vi "Main v0.86.vi"() -> ()   [LabVIEW 2017]
doc: "v0.85:\n- Counts for rejects and total\n\nv0.5:\n\n- Added Reject to Manual Mode\n- Send reject pallet cluster during manual mode\n- Run continuous manual happens only when no error has occured"
uses:
  Controls/Main Tabs.ctl
  Controls/Auto.ctl
  RT/Controls/Auto Delays.ctl
  RT/Controls/Auto Times.ctl
  Controls/UI Data.ctl
  support/Message Queue/Enqueue Message (Single).vi
  <vilib>/Utility/error.llb/Error Cluster From Error Code.vi
  <vilib>/ErrorRing/Error Ring.xnode
  support/Message Queue/Message Queue.lvlib
  support/User Event - Stop/User Event - Stop.lvlib
panel:
  in  "Reject Pallets":T1
  out "Date-Time":string caption="Dip-Tube Assembly Automation (HMI) v0.85"
  out "Main Tab":T2
  in  "Autocycle":T3
  in  "Manual":bool
  in  "Parameters":bool
  in  "Maintenance":bool
  in  "Save Para":bool
  in  "Home Para":bool
  in  "ParaTab":T4(tab)
  in  "StopperRearDelay":dbl format="%#.2f"
  in  "StopperFrontDelay":dbl format="%#.2f"
  in  "MaxAlarms":dbl caption="Max Alarms in 1 Minute" format="%#.2f"
  in  "MaxConsecutive":dbl caption="Max Consecutive Alarms" format="%#.2f"
  in  "Gate Close Delay":dbl format="%#.2f"
  in  "Gate Open Delay":dbl format="%#.2f"
  in  "BF Off Delay":dbl format="%#.2f"
  in  "BF On Delay":dbl format="%#.2f"
  in  "DelayAfterReject":dbl format="%#.2f"
  in  "MeasurementTime":dbl format="%#.2f"
  in  "DelayAfterMesFront":dbl format="%#.2f"
  in  "DelayAfterCut":dbl format="%#.2f"
  in  "DelayAfterCutClamp":dbl format="%#.2f"
  in  "DelayAfterInsClamp":dbl format="%#.2f"
  in  "DelayToClose":dbl format="%#.2f"
  in  "DelayToOpen":dbl format="%#.2f"
  in  "DelayAfterInsertion":dbl format="%#.2f"
  in  "DelayBeforeInsertion":dbl format="%#.2f"
  in  "AgitatorUpTime":dbl format="%#.2f"
  in  "AgitatorDownTime":dbl format="%#.2f"
  out "OEE":dbl format="%#.1f"
  out "QUA":dbl=100.0 min=0.0 max=100.0 step=0.1
  in  "Ideal Time":dbl=2.0 min=0.0 max=100.0 step=0.1
  in  "AVL":dbl=100.0 min=0.0 max=100.0 step=0.1
  out "Rejects":u32
  in  "Reset MCount":bool
  in  "Enable BF?":bool
  in  "Enable Agitate?":bool
  in  "Enable Reject?":bool
  in  "Toggle Motor":bool
  in  "Continuous?":bool
  in  "Enable Measure?":bool
  in  "Enable Index?":bool
  in  "Enable PF?":bool
  in  "Auto Delays":T5={"Agitator Delays"=[400, 250], "TF Delays"=[700, 800, 2], "Insertion Delays"=[100, 500], "Cutting Delays"=[300, 300, 100], "PF Delays"=[250, 30000], "Measur. Delays"=[500.0, 188.9, 1.0], "Reject Delays"=[500], "BF Delays"=[1000, 1000]}
  in  "Enable Cutting?":bool
  in  "Enable Insertion?":bool
  in  "Run Manual":bool
  in  "Enable TF?":bool
  in  "Home Manual":bool
  out "Status":T7
  out "Measurements":T8 {"Height 1" format="%#.2f"; "Height 2" format="%#.2f"; "Height 3" format="%#.2f"; "Height 4" format="%#.2f"}
  out "Output Count":u32 caption="Output\nCount"
  out "PRF":dbl=100.0 min=0.0 max=100.0 step=0.1
  in  "All IO":bool
  in  "Stats":bool
  in  "Home AC":bool
  out "Status":string
  out "Count":dbl format="%06.0f"
  out "Count 3":dbl caption="Cycle Time" format="%0.2f"
  out "Count 2":dbl caption="Rejects" format="%06.0f"
  in  "Statuses":string[][](table)
  in  "Exit":bool
  # "Vision Harmony Dip-Tube Assembly Automation"
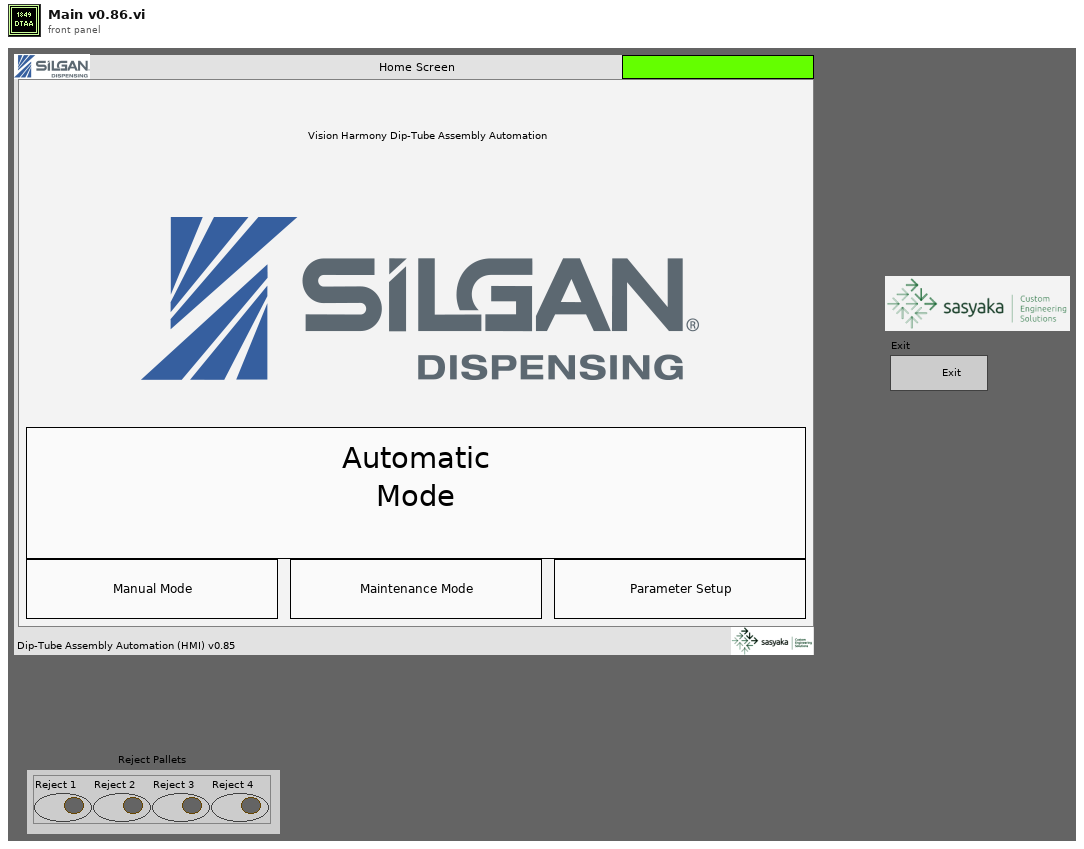
[diagram p1: front panel]
types:
  T1 = cluster{"Reject 1":bool, "Reject 2":bool, "Reject 3":bool, "Reject 4":bool}
  T2 = typedef "Main Tabs.ctl" = enum32{"Home Screen", "Parameter Setup", "Manual Mode", "Autocycle"}
  T3 = typedef "Auto.ctl" = bool
  T4 = enum32{"General & Indexing", "Bowl Feeder & Pump Conveyor", "Cutting, Measurement & Rejection", "Tube Feeder & Insertion"}
  T5 = typedef "Auto Delays.ctl" = cluster{"Agitator Delays":u32[], "TF Delays":u32[], "Insertion Delays":u32[], "Cutting Delays":u32[], "PF Delays":u32[], "Measur. Delays":dbl[], "Reject Delays":u32[], "BF Delays":u32[]}
  T6 = typedef "Auto Times.ctl" = cluster{"Index Time":u32, "TF Time":u32, "Insertion Time":u32, "Cutting Time":u32, "PF Time":u32, "Meas. Time":u32, "Reject Time":u32}
  T7 = cluster{"Auto Times":T6, "error out":errorcluster}
  T8 = cluster{"Height 1":dbl, "Height 2":dbl, "Height 3":dbl, "Height 4":dbl}
  T9 = typedef "UI Data.ctl" = cluster{"Main Tab":refnum<vi>}
  T10 = typedef "Message Queue.lvlib/All Message Queues.ctl" = cluster{"UI":refnum<queue>}
  T11 = enum8{"Enabled", "Disabled", "Disabled and Grayed Out"}
  T12 = cluster{"Auto Times":T6, "Results":cluster{"Measurements":cluster{"1":dbl, "2":dbl, "3":dbl, "4":dbl}, "Reject Pallets":cluster{"Reject 1":bool, "Reject 2":bool, "Reject 3":bool, "Reject 4":bool}}, "OutputCount":u32, "error out":errorcluster}
  T13 = cluster{"Auto Delays":T5, "Reject Pallets":cluster{"Reject 1":bool, "Reject 2":bool, "Reject 3":bool, "Reject 4":bool}}
  T14 = cluster{"Measurements":cluster{"1":dbl, "2":dbl, "3":dbl, "4":dbl}, "Reject Pallets":cluster{"Reject 1":bool, "Reject 2":bool, "Reject 3":bool, "Reject 4":bool}}
  T15 = cluster{"AVL":dbl, "PRF":dbl, "QUA":dbl, "OEE":dbl}
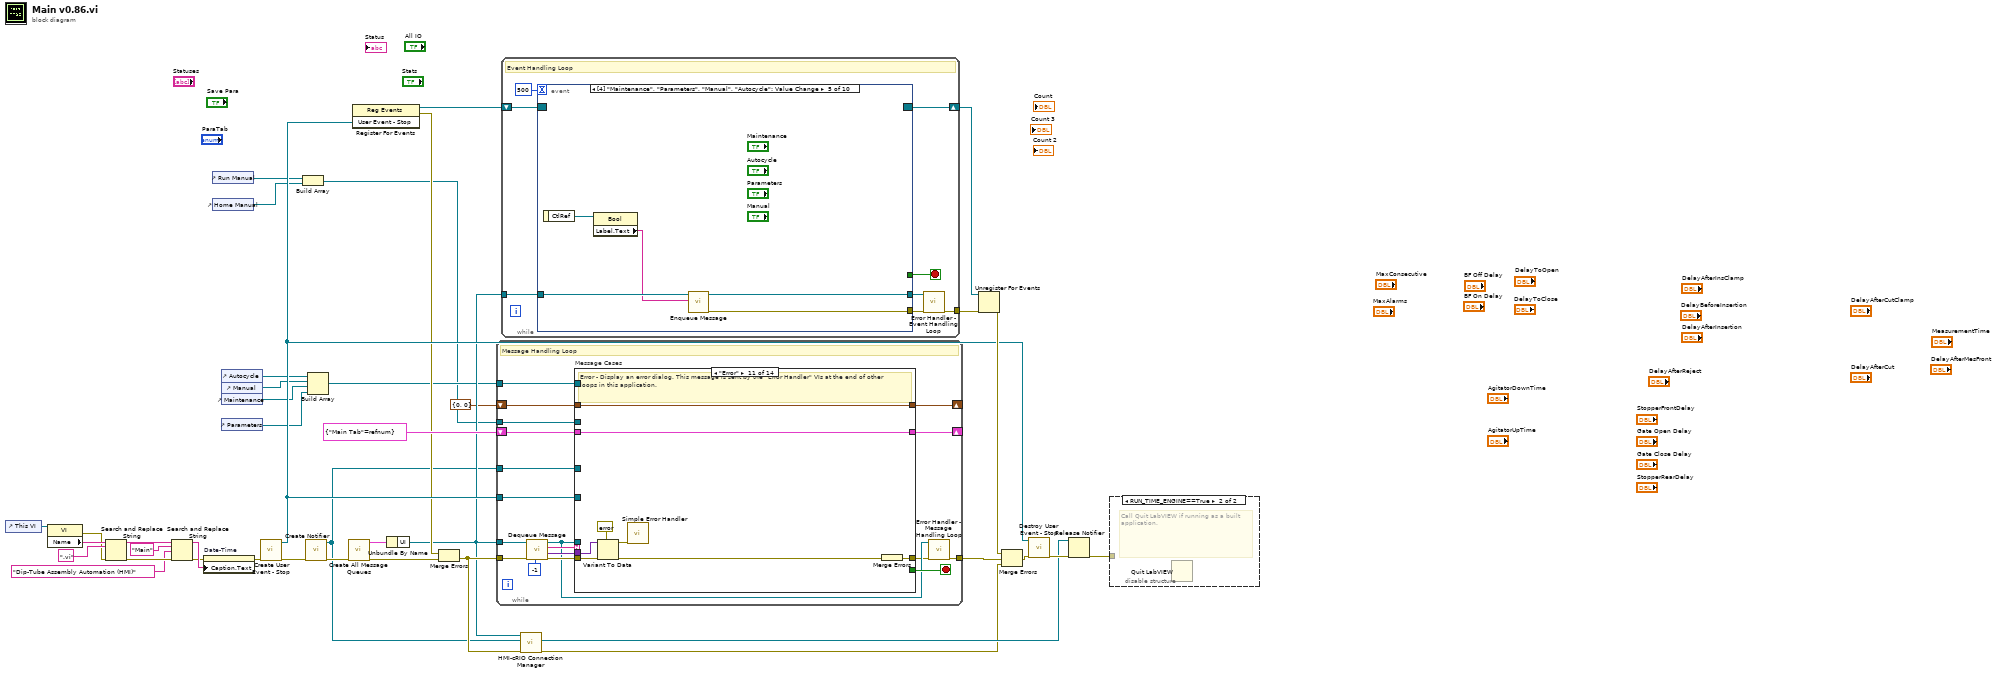
[diagram p0: block diagram]
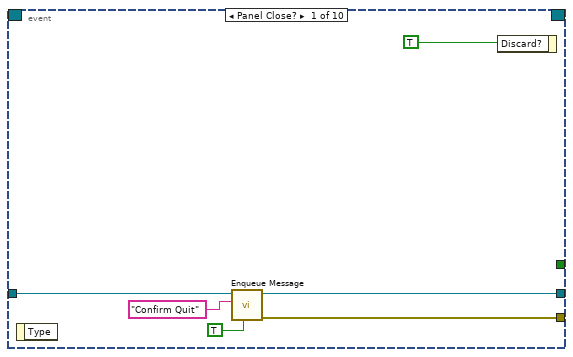
[diagram p2: hidden frame]
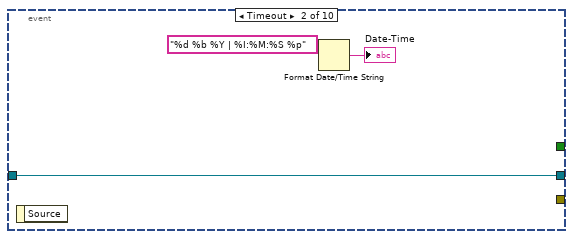
[diagram p3: hidden frame]
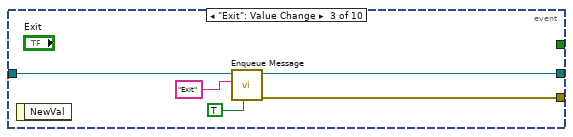
[diagram p4: hidden frame]
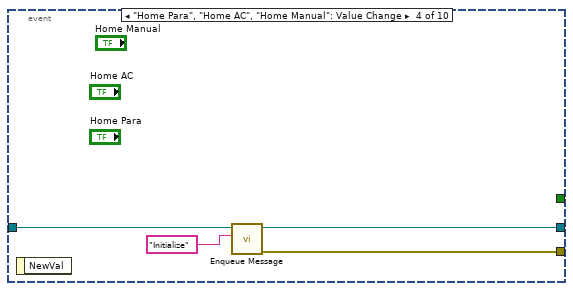
[diagram p5: hidden frame]
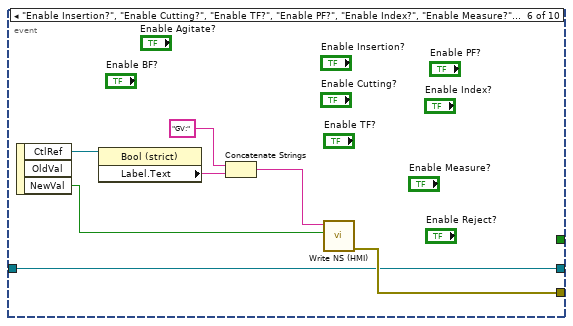
[diagram p6: hidden frame]
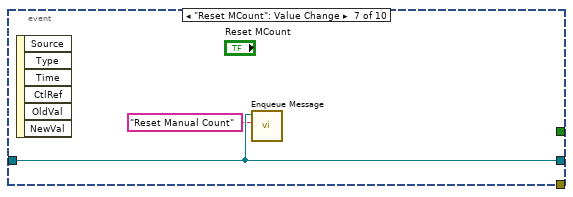
[diagram p7: hidden frame]
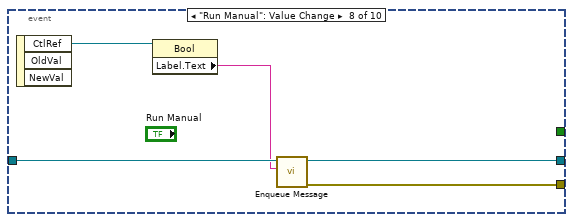
[diagram p8: hidden frame]
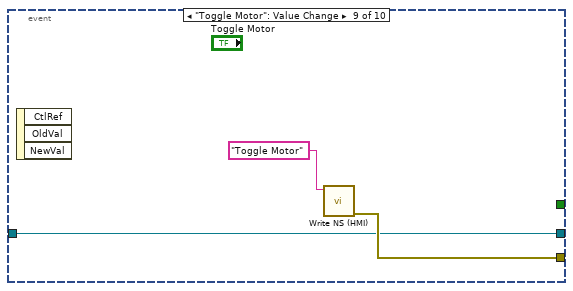
[diagram p9: hidden frame]
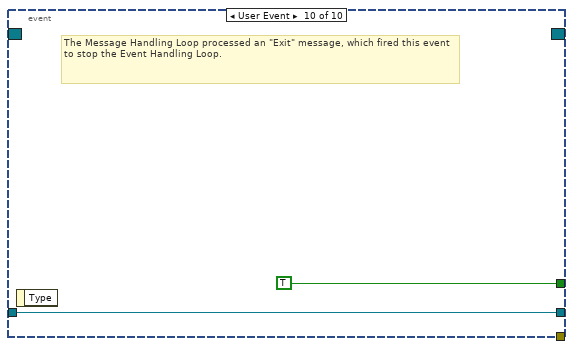
[diagram p10: hidden frame]
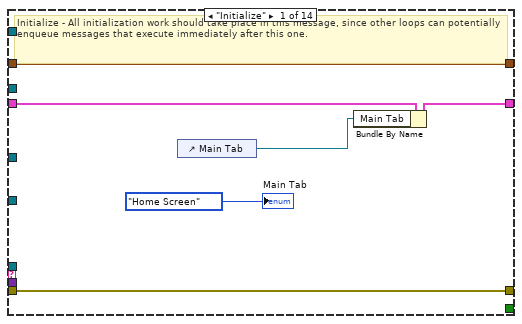
[diagram p11: hidden frame]
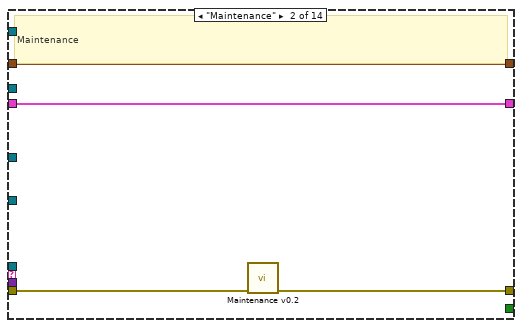
[diagram p12: hidden frame]
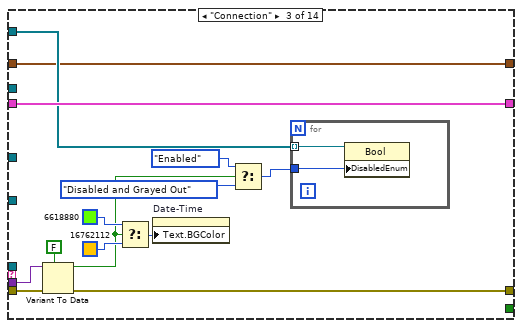
[diagram p13: hidden frame]
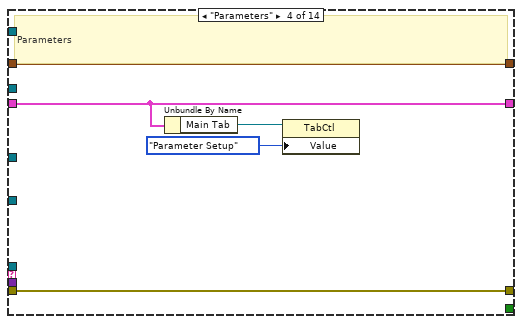
[diagram p14: hidden frame]
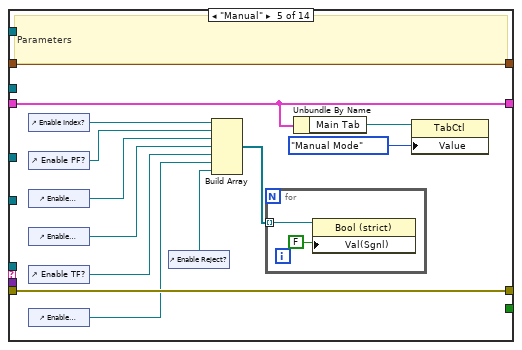
[diagram p15: hidden frame]
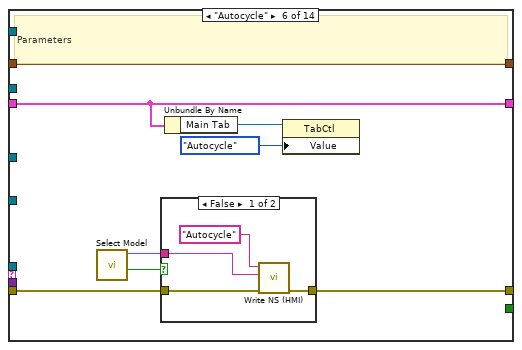
[diagram p16: hidden frame]
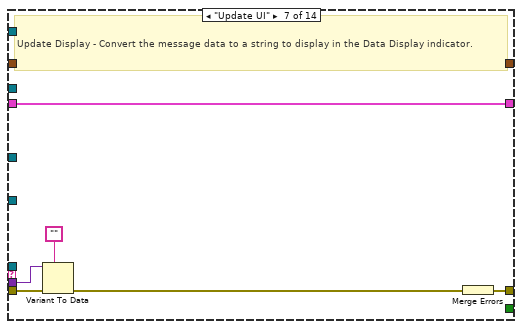
[diagram p18: hidden frame]
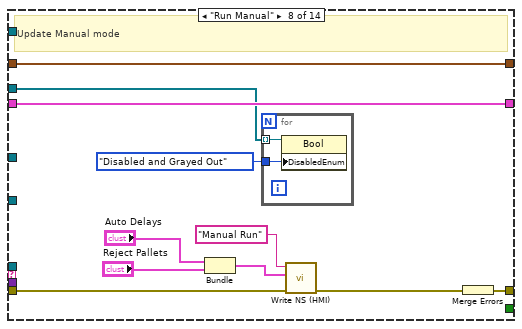
[diagram p19: hidden frame]
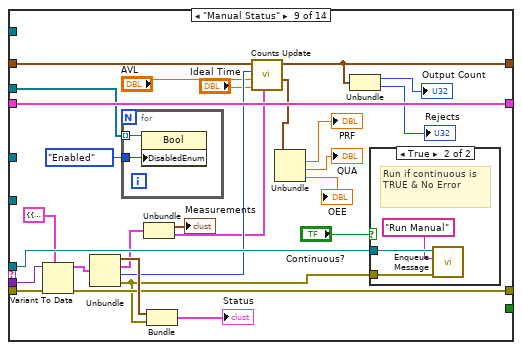
[diagram p20: hidden frame]
diagram:
  n1 = control-ref of="This VI"() -> (w9:refnum<vi>)
  n2 = property class="VI"(reference=w9) -> (error out=w8:errorcluster, "Name"=w15:string)  [unwired: 1 in, 1 out]
  n3 = Search and Replace String(input string=w15, search string=".vi", error in=w8) -> (result string=w13:string, error out=w12:errorcluster)  [unwired: 5 in, 2 out]
  n4 = Search and Replace String(input string=w13, search string="Main", replace string="Dip-Tube Assembly Automation (HMI)" ("replace string (\"\")"), error in=w12) -> (result string=w7:string, error out=w6:errorcluster)  [unwired: 4 in, 2 out]
  n5 = property on="Date-Time" class="Str"(error in=w6, "Caption.Text"=w7) -> (error out=w5:errorcluster)  [unwired: 1 in, 1 out]
  n6 = control-ref of="Run Manual"() -> (w4:refnum<vi>)
  n7 = control-ref of="Home Manual"() -> (w3:refnum<vi>)
  n8 = control-ref of="Autocycle"() -> (w20:refnum<vi>)
  n9 = control-ref of="Manual"() -> (w19:refnum<vi>)
  n10 = control-ref of="Maintenance"() -> (w18:refnum<vi>)
  n11 = control-ref of="Parameters"() -> (w17:refnum<vi>)
  n12 = call "Create User Event - Stop.vi"("error in (no error)"=w5) -> ("error out"=w27:errorcluster, "User Event - Stop"=w31:refnum<user-event>)  [unwired: 9 in]
  n13 = Build Array(w4, w3) -> (w2:refnum<vi>[])
  n14 = call "Create Notifier.vi"("error in (no error)"=w27) -> ("error out"=w26:errorcluster, "notifier out"=w21:refnum<notifier>)  [unwired: 9 in]
  n15 = Build Array(w20, w19, w18, w17) -> (w16:refnum<vi>[])
  n16 = call "Create All Message Queues.vi"("error in (no error)"=w26) -> ("error out"=w40:errorcluster, "Message Queues out"=w39:T10)  [unwired: 9 in]
  n17 = register-events(w31) -> (reference out=w32:refnum<event-registration>, error out=w30:errorcluster)  [unwired: 2 in]
  n18 = Unbundle By Name(w39) -> ("UI"=w28:refnum<queue>)
  n19 = Merge Errors(w30, w40) -> (w29:errorcluster)
  n20 = while {
    tunnel: w28 -> [w50]
    shift-right: [w57] -> _
    shift-left: T9 {"Main Tab"=refnum} ("Data Cluster") -> [w58]
    tunnel: w31 -> [w55]
    tunnel: w29 -> [w54]
    tunnel: [w48] -> w38
    tunnel: w21 -> [w45]
    tunnel: w16 -> [w44]
    tunnel: w2 -> [w43]
    shift-right: [w41] -> _
    shift-left: cluster{"OutputCount":u32, "RejectCount":u32} {"OutputCount"=0, "RejectCount"=0} -> [w42]
    stop <- w56 stop-if-true
    # "Message Handling Loop"
    n21 = call "Dequeue Message.vi"("timeout"=-1, "error in (no error)"=w54, "Message Queue"=w50) -> ("error out"=w53:errorcluster, "Message Data"=w51:variant, "Message"=w52:string, "dup Message Queue"=w49:refnum<queue>)  [unwired: 5 in]
    n22 = case "Message Cases" shown="\"Error\"" w52 {
      selector: w52 -> [_ _ _ _ _ _ _ _ _ _ _ _ _ w206]
      tunnel: w49 -> [_ _ _ _ _ _ _ _ w155 _ _ w185 w204 _]
      tunnel: w53 -> [w64 w67 w80 w89 w102 w108 w122 w132 w163 w173 w181 w189 w197 _]
      tunnel: [w64 w66 w79 w89 w102 w107 w123 w134 w154 w173 w175 w187 w200 w207] -> w47
      tunnel: w58 -> [w63 w68 w82 w88 w101 w112 w124 w135 w164 w172 w180 w188 w203 w208]
      tunnel: [w62 w68 w82 w88 w101 w112 w124 w135 w164 w172 w180 w188 w203 w208] -> w57
      tunnel: [_ _ _ _ _ _ _ _ _ _ _ _ TRUE _] -> w56
      tunnel: w51 -> [_ _ w78 _ _ _ w121 _ w162 _ w179 _ w194 _]
      tunnel: w55 -> [_ _ _ _ _ _ _ _ _ _ _ _ w199 _]
      tunnel: w45 -> [_ _ _ _ _ _ _ _ _ _ _ _ w193 _]
      tunnel: w44 -> [_ _ w74 _ _ _ _ _ _ _ _ _ _ _]
      tunnel: w43 -> [_ _ _ _ _ _ _ w129 w160 _ _ _ _ _]
      tunnel: w42 -> [w59 w65 w69 w85 w90 w109 w118 w125 w153 _ w174 w182 w190 w205]
      tunnel: [w59 w65 w69 w85 w90 w109 w118 w125 w146 cluster{"OutputCount":u32, "RejectCount":u32} {"OutputCount"=0, "RejectCount"=0} w174 w182 w190 w205] -> w41
      frame "Initialize" {
        # "Initialize - All initialization work should take place in this message, since other loops can potentially enqueue messages that execute immediately after this one."
        n23 = control-ref of="Main Tab"() -> (w61:refnum<vi>)
        n24 = Bundle By Name(cluster=w63, "Main Tab"=w61) -> (w62:T9)
        "Main Tab" <- Main_Tabs."Home Screen" ("Main Tab")
      }
      frame "Maintenance" {
        # "Maintenance"
        n25 = call "Maintenance v0.2.vi"("Error In"=w67) -> ("Error out"=w66:errorcluster)  [unwired: 10 in]
      }
      frame "Connection" {
        n26 = Variant To Data(error in=w80, type=FALSE, Variant=w78) -> (data=w73:bool, error out=w79:errorcluster)
        n27 = Select(t=u32 6618880 ("Text.Text Colors:BG Color"), s=w73, f=u32 16762112 ("Text.Text Colors:BG Color")) -> (s? t:f=w75:u32)
        n28 = property on="Date-Time" class="Str"("Text.BGColor"=w75) -> ()  [unwired: 2 in, 2 out]
        n29 = Select(t=T11."Enabled" ("Disabled"), s=w73, f=T11."Disabled and Grayed Out") -> (s? t:f=w71:T11)
        n30 = for {
          tunnel: w74 -> [w84] mode=indexing
          tunnel: w71 -> [w83]
          n31 = property class="Bool"(reference=w84, "DisabledEnum"=w83) -> ()  [unwired: 1 in, 2 out]
        }
      }
      frame "Parameters" {
        # "Parameters"
        n32 = Unbundle By Name(w88) -> ("Main Tab"=w87:refnum<vi>)
        n33 = property class="TabCtl"(reference=w87, "Value"=Main_Tabs."Parameter Setup" ("Main Tab")) -> ()  [unwired: 1 in, 2 out]
      }
      frame "Manual" {
        # "Parameters"
        n34 = control-ref of="Enable Index?"() -> (w98:refnum<vi>)
        n35 = control-ref of="Enable PF?"() -> (w97:refnum<vi>)
        n36 = control-ref of="Enable Cutting?"() -> (w96:refnum<vi>)
        n37 = control-ref of="Enable Insertion?"() -> (w95:refnum<vi>)
        n38 = control-ref of="Enable TF?"() -> (w94:refnum<vi>)
        n39 = control-ref of="Enable Measure?"() -> (w92:refnum<vi>)
        n40 = control-ref of="Enable Reject?"() -> (w91:refnum<vi>)
        n41 = Build Array(w98, w97, w96, w95, w94, w92, w91) -> (w93:refnum<vi>[])
        n42 = for {
          tunnel: w93 -> [w104] mode=indexing
          n43 = property class="Bool (strict)"(reference=w104, "Val(Sgnl)"=FALSE ("Value (Signaling)")) -> ()  [unwired: 1 in, 2 out]
        }
        n44 = Unbundle By Name(w101) -> ("Main Tab"=w100:refnum<vi>)
        n45 = property class="TabCtl"(reference=w100, "Value"=Main_Tabs."Manual Mode" ("Main Tab")) -> ()  [unwired: 1 in, 2 out]
      }
      frame "Autocycle" {
        # "Parameters"
        n46 = call "Select Model.vi"() -> ("Cancel out"=w105:bool, "Model out"=w106:string)  [unwired: 10 in]
        n47 = case shown="False" w105 {
          tunnel: w108 -> [w115 w117]
          tunnel: [w114 w117] -> w107
          tunnel: w106 -> [w113 _]
          frame False {
            n48 = call "Write NS (HMI).vi"("error in (no error)"=w115, "Message Data"=w113, "Message"="Autocycle") -> ("error out"=w114:errorcluster)  [unwired: 8 in]
          }
          frame True {
          }
        }
        n49 = Unbundle By Name(w112) -> ("Main Tab"=w111:refnum<vi>)
        n50 = property class="TabCtl"(reference=w111, "Value"=Main_Tabs."Autocycle" ("Main Tab")) -> ()  [unwired: 1 in, 2 out]
      }
      frame "Update UI" {
        # "Update Display - Convert the message data to a string to display in the Data Display indicator."
        n51 = Variant To Data(error in=w122, type="", Variant=w121) -> (error out=w119:errorcluster)  [unwired: 1 out]
        n52 = Merge Errors(w119) -> (w123:errorcluster)
      }
      frame "Run Manual" {
        # "Update Manual mode"
        n53 = Bundle("Auto Delays"="Auto Delays", "Reject Pallets"="Reject Pallets") -> (w126:T13)  [unwired: 1 in]
        n54 = for {
          tunnel: w129 -> [w137] mode=indexing
          tunnel: T11."Disabled and Grayed Out" ("Disabled") -> [w136]
          n55 = property class="Bool"(reference=w137, "DisabledEnum"=w136) -> ()  [unwired: 1 in, 2 out]
        }
        n56 = call "Write NS (HMI).vi"("error in (no error)"=w132, "Message Data"=w126, "Message"="Manual Run") -> ("error out"=w131:errorcluster)  [unwired: 8 in]
        n57 = Merge Errors(w131) -> (w134:errorcluster)
      }
      frame "Manual Status" {
        n58 = Variant To Data(error in=w163, type=T12 {"Auto Times"={"Index Time"=0, "TF Time"=0, "Insertion Time"=0, "Cutting Time"=0, "PF Time"=0, "Meas. Time"=0, "Reject Time"=0}, "Results"={"Measurements"={"1"=0.0, "2"=0.0, "3"=0.0, "4"=0.0}, "Reject Pallets"={"Reject 1"=FALSE, "Reject 2"=FALSE, "Reject 3"=FALSE, "Reject 4"=FALSE}}, "OutputCount"=0, "error out"={"status"=FALSE, "code"=0, "source"=""}} ("cluster"), Variant=w162) -> (data=w159:T12, error out=w154:errorcluster)
        n59 = Unbundle(w159) -> ("Auto Times"=w158:T6, "Results"=w150:T14, "OutputCount"=w148:u32, "error out"=w152:errorcluster)
        n60 = for {
          tunnel: w160 -> [w169] mode=indexing
          tunnel: T11."Enabled" ("Disabled") -> [w168]
          n61 = property class="Bool"(reference=w169, "DisabledEnum"=w168) -> ()  [unwired: 1 in, 2 out]
        }
        n62 = Unbundle(w150) -> ("Measurements"=→"Measurements":cluster{"1":dbl, "2":dbl, "3":dbl, "4":dbl}, "Reject Pallets"=w147:T1)
        n63 = Bundle("Auto Times"=w158, "error out"=w152) -> (→"Status":T7)  [unwired: 1 in]
        n64 = call "Counts Update.vi"("Reject Pallets"=w147, "Desired Cycle Time"="Ideal Time", "AVL"="AVL", "OutputCount"=w148, "Counts in"=w153) -> ("OEE"=w141:T15, "Counts out"=w146:cluster{"OutputCount":u32, "RejectCount":u32})  [unwired: 5 in]
        n65 = Unbundle(w141) -> ("PRF"=→"PRF":dbl, "QUA"=→"QUA":dbl, "OEE"=→"OEE":dbl)  [unwired: 1 out]
        n66 = Unbundle(w146) -> ("OutputCount"=→"Output Count":u32, "RejectCount"=→"Rejects":u32)
        n67 = case shown="True" "Continuous?" {
          tunnel: w155 -> [_ w167]
          tunnel: w152 -> [_ w166]
          frame False {
          }
          frame True {
            # "Run if continuous is TRUE & No Error"
            n68 = call-poly "Enqueue Message.vi"("error in (no error)"=w166, "Message"="Run Manual", "Message Queue"=w167) -> ()  [unwired: 7 in, 2 out]
          }
        }
      }
      frame "Reset Manual Count" {
        w170 = u32 0 ("Rejects")
        n69 = local write "Output Count"(w170) -> ()
        n70 = local write "Rejects"(w170) -> ()
      }
      frame "Error" {
        # "Error - Display an error dialog. This message is sent by the \"Error Handler\" VIs at the end of other loops in this application."
        n71 = Variant To Data(error in=w181, type=errorcluster {"status"=FALSE, "code"=0, "source"=""} ("error constant"), Variant=w179) -> (data=w177:errorcluster, error out=w176:errorcluster)
        n72 = call <vilib>:"Simple Error Handler.vi"("error in (no error)"=w177) -> ()  [unwired: 4 in, 5 out]
        n73 = Merge Errors(w176) -> (w175:errorcluster)
      }
      frame "Confirm Quit" {
        # "Confirm Quit - Message that can confirm whether or not the user wants to exit the application."
        n74 = call-poly "Enqueue Message.vi"("Priority Message? (F)"=TRUE, "error in (no error)"=w189, "Message"="Exit", "Message Queue"=w185) -> ("error out"=w186:errorcluster)  [unwired: 6 in, 1 out]
        n75 = Merge Errors(w186) -> (w187:errorcluster)
      }
      frame "Exit" {
        # "Stop the VI"
        # "Release the message queue reference"
        # "Exit - Exit the application."
        n76 = Variant To Data(type=errorcluster {"status"=FALSE, "code"=0, "source"=""} ("error constant"), Variant=w194) -> (data=w195:errorcluster)  [unwired: 1 in, 1 out]
        n77 = call <vilib>:"Simple Error Handler.vi"("error in (no error)"=w195) -> ()  [unwired: 4 in, 5 out]
        n78 = Send Notification(notification=TRUE, notifier=w193) -> (error out=w191:errorcluster)  [unwired: 1 in, 1 out]
        n79 = call "Fire User Event - Stop.vi"("User Event - Stop"=w199) -> ("error out"=w198:errorcluster)  [unwired: 10 in]
        n80 = Release Queue(queue=w204, error in (no error)=w197) -> (error out=w201:errorcluster)  [unwired: 1 in, 2 out]
        n81 = Merge Errors(w191, w198, w201) -> (w200:errorcluster)
      }
      frame Default {
        # "'Default' case only runs if there is a message that isn't defined in any of the other cases.  Output a programming error."
        n82 = xnode "Error Ring"("parameter 0"=w206) -> ("error out"=w207:errorcluster)
      }
    }
    n83 = call "Error Handler - Message Handling Loop.vi"("error in (no error)"=w47, "Message Queue"=w49) -> ("dup error in"=w48:errorcluster)  [unwired: 8 in, 1 out]
  }
  n84 = while {
    tunnel: w28 -> [w223]
    shift-right: [w221] -> w35
    shift-left: w32 -> [w222]
    tunnel: [w217] -> w33
    stop <- w219 stop-if-true
    # "Event Handling Loop"
    n85 = event shown="[4] \"Maintenance\", \"Parameters\", \"Manual\", \"Autocycle\": Value Change" {
      selector: w222 -> [_ _ _ _ _ _ _ _ _ _]
      dyn-events: [_ _ _ _ _ _ _ _ _ _] -> w221
      timeout: 500 -> [_ _ _ _ _ _ _ _ _ _]
      tunnel: [_ _ _ _ _ _ _ _ _ TRUE ("Discard?")] -> w219
      tunnel: w223 -> [w228 w232 w237 w241 w246 w251 w255 w260 w262 w265]
      tunnel: [w227 _ w236 w240 w245 w252 _ w258 w263 _] -> w220
      tunnel: [w226 w232 w235 w239 w244 w251 w255 w259 w262 w265] -> w218
      event Panel Close? {
        n86 = event-data() -> ()  [unwired: 1 in, 1 out]
        n87 = call-poly "Enqueue Message.vi"("Priority Message? (F)"=TRUE, "Message"="Confirm Quit", "Message Queue"=w228) -> ("error out"=w227:errorcluster, "dup Message Queue"=w226:refnum<queue>)  [unwired: 7 in]
        n88 = event-data("Discard?"=TRUE) -> ()  [unwired: 1 in, 1 out]
      }
      event Timeout {
        n89 = event-data() -> ()  [unwired: 1 in, 1 out]
        n90 = Format Date/Time String(time format string (%c)="%d %b %Y | %I:%M:%S %p") -> (date/time string=→"Date-Time":string)  [unwired: 2 in]
      }
      event "Exit": Value Change {
        n91 = event-data() -> ()  [unwired: 1 in, 1 out]
        n92 = call-poly "Enqueue Message.vi"("Priority Message? (F)"=TRUE, "Message"="Exit", "Message Queue"=w237) -> ("error out"=w236:errorcluster, "dup Message Queue"=w235:refnum<queue>)  [unwired: 7 in]
      }
      event "Home Para", "Home AC", "Home Manual": Value Change {
        n93 = event-data() -> ()  [unwired: 1 in, 1 out]
        n94 = call-poly "Enqueue Message.vi"("Message"="Initialize", "Message Queue"=w241) -> ("error out"=w240:errorcluster, "dup Message Queue"=w239:refnum<queue>)  [unwired: 8 in]
      }
      event "Maintenance", "Parameters", "Manual": Value Change {
        n95 = event-data() -> ("CtlRef"=w243:refnum<vi>)  [unwired: 1 in]
        n96 = property class="Bool"(reference=w243) -> ("Label.Text"=w242:string)  [unwired: 1 in, 2 out]
        n97 = call-poly "Enqueue Message.vi"("Message"=w242, "Message Queue"=w246) -> ("error out"=w245:errorcluster, "dup Message Queue"=w244:refnum<queue>)  [unwired: 8 in]
      }
      event "Enable Insertion?", "Enable Cutting?", "Enable TF?", "Enable PF?", "Enable Index?", "Enable Measure?", "Enable Reject?", "Enable Agitate?", "Enable BF?": Value Change {
        n98 = event-data() -> ("CtlRef"=w253:refnum<vi>, "NewVal"=w247:bool)  [unwired: 1 in, 1 out]
        n99 = property class="Bool (strict)"(reference=w253) -> ("Label.Text"=w250:string)  [unwired: 1 in, 2 out]
        n100 = Concatenate Strings("GV:" ("string"), w250) -> (w248:string)
        n101 = call "Write NS (HMI).vi"("Message Data"=w247, "Message"=w248) -> ("error out"=w252:errorcluster)  [unwired: 9 in]
      }
      event "Reset MCount": Value Change {
        n102 = event-data() -> ()  [unwired: 1 in, 6 out]
        n103 = call-poly "Enqueue Message.vi"("Message"="Reset Manual Count", "Message Queue"=w255) -> ()  [unwired: 8 in, 2 out]
      }
      event "Run Manual": Value Change {
        n104 = event-data() -> ("CtlRef"=w257:refnum<vi>)  [unwired: 1 in, 2 out]
        n105 = property class="Bool"(reference=w257) -> ("Label.Text"=w256:string)  [unwired: 1 in, 2 out]
        n106 = call-poly "Enqueue Message.vi"("Message"=w256, "Message Queue"=w260) -> ("error out"=w258:errorcluster, "dup Message Queue"=w259:refnum<queue>)  [unwired: 8 in]
      }
      event "Toggle Motor": Value Change {
        n107 = event-data() -> ()  [unwired: 1 in, 3 out]
        n108 = call "Write NS (HMI).vi"("Message"="Toggle Motor") -> ("error out"=w263:errorcluster)  [unwired: 10 in]
      }
      event User Event {
        # "The Message Handling Loop processed an \"Exit\" message, which fired this event to stop the Event Handling Loop."
        n109 = event-data() -> ()  [unwired: 1 in, 1 out]
      }
    }
    n110 = call "Error Handler - Event Handling Loop.vi"("error in (no error)"=w220, "Message Queue"=w218) -> ("dup error in"=w217:errorcluster)  [unwired: 8 in, 1 out]
  }
  n111 = call "HMI-cRIO Connection Manager.vi"("error in"=w29, "notifier in"=w21, "Queue in"=w28) -> ("error out"=w22:errorcluster, "Notifier out"=w23:refnum<notifier>)  [unwired: 7 in]
  n112 = Unregister For Events(event registration refnum=w35, error in=w33) -> (error out=w36:errorcluster)
  n113 = Merge Errors(w36, w38, w22) -> (w37:errorcluster)
  n114 = call "Destroy User Event - Stop.vi"("error in (no error)"=w37, "User Event - Stop"=w31) -> ("error out"=w25:errorcluster)  [unwired: 9 in]
  n115 = Release Notifier(notifier=w23, error in (no error)=w25) -> (error out=w24:errorcluster)  [unwired: 1 in, 2 out]
  n116 = disable-structure shown="RUN_TIME_ENGINE==True" {
    disable-tunnel: w24 -> [_ _]
    frame condition #0 (active) {
    }
    frame condition #1 {
      # "Call Quit LabVIEW if running as a built application."
      n117 = Quit LabVIEW() -> ()  [unwired: 1 in]
    }
  }
